vi "Online Spectrogram Monitoring (Sound Card).vi"() -> ()   [LabVIEW 2023]
doc: "This example shows how to configure a sound card device, continuously acquire sound data, and compute the real-time STFT spectrogram with the TFA Online STFT Spectrogram VI.\n\n<b>Instructions:</b>\n1) Run this VI.\n2) Speak or whistle into the microphone.\n3) Observe the <b>Spectrogram</b> to see the frequencies that this VI detects.\n4) Browse the Block Diagram of this example to learn how to configure the charts."
uses:
  <vilib>/sound2/lvsound2.llb/Sound Data Format.ctl
  <vilib>/Analysis/baseanly.llb/Mean (DBL).vi
  <vilib>/sound2/lvsound2.llb/Sound Input Read (DBL).vi
  <vilib>/addons/Time Frequency Analysis/Spectrogram.llb/TFA Online STFT Spectrogram (Real).vi
  <vilib>/addons/Time Frequency Analysis/_control.llb/TFA Configure Spectrogram Indicator (Predefined Color Table).vi
  <vilib>/addons/_Advanced Signal Processing/NI_AdvSigProcTFA.lvlib
  <vilib>/Analysis/NI_AALBase.lvlib
panel:
  out "aspt-left-top":bool
  in  "dB on?(F)":bool
  in  "Stop":bool
  out "Signal":dbl[](graph)
  out "Spectrogram":dbl[][](graph)
  # "Overview: Shows how to configure a sound card device, continuously acquire sound data, and compute the real-time STFT spectrogram with the TFA Online STFT Spectrogram VI.\nRequirements: LabVIEW Full Development System, Advanced Signal Processing Toolkit, microphone\nInstructions: \n1. Run this VI.\n2. Speak or whistle into the microphone.\n3. Observe the Spectrogram to see the frequencies that this VI detects.\n4. Browse the block diagram of this example to learn how to configure the charts.\n5. Click Stop to stop the VI."
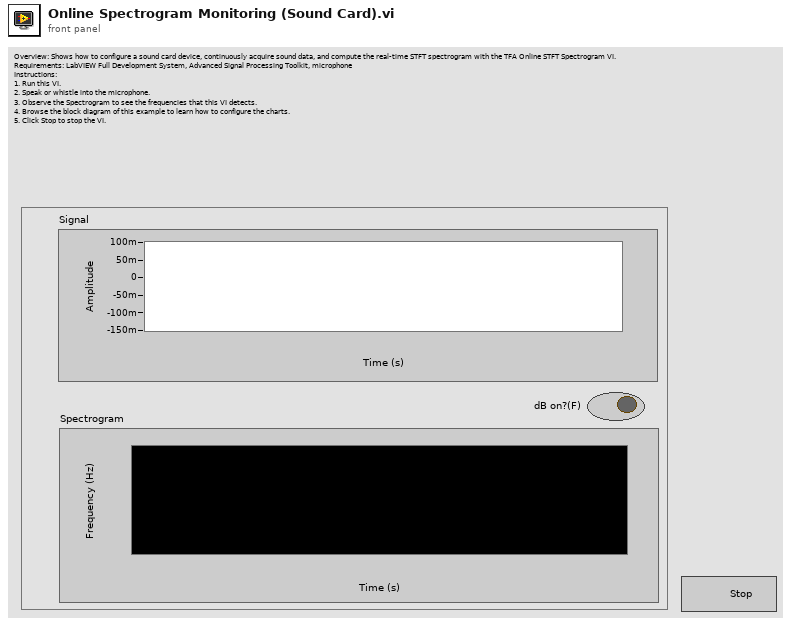
[diagram p1: front panel]
types:
  T1 = typedef "Sound Data Format.ctl" = cluster{"sample rate (S/s)":dbl, "number of channels":i32, "bits per sample":i32}
  T2 = typedef "Sound Input Task ID.ctl" = u32
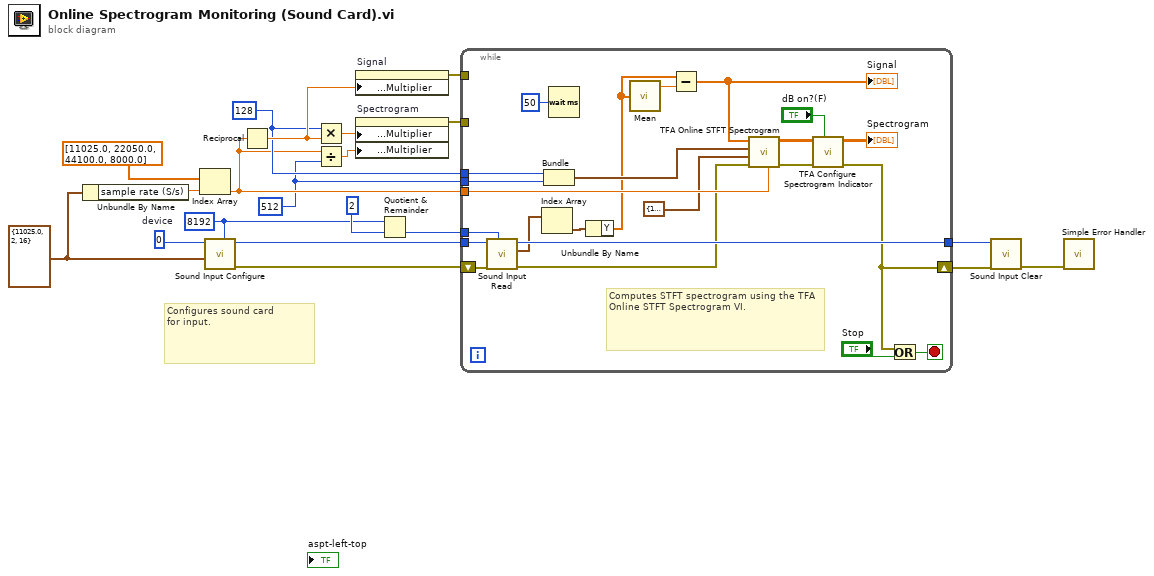
[diagram p0: block diagram]
diagram:
  w8 = T1 {"sample rate (S/s)"=11025.0, "number of channels"=2, "bits per sample"=16} ("sound format")
  w9 = 512 ("FFT block size")
  w12 = 128 ("Step size")
  w4 = 8192 ("Buffer Size")
  w20 = u32 0  # device
  # "Configures sound card\nfor input."
  n1 = Unbundle By Name(w8) -> ("sample rate (S/s)"=w17:dbl)
  n2 = Index Array(array=dbl[] [11025.0, 22050.0, 44100.0, 8000.0], index=w17) -> (element=w10:dbl)
  n3 = call <vilib>:"Sound Input Configure.vi"("number of samples/ch"=w4, "sound format"=w8, "device ID"=w20) -> ("error out"=w6:errorcluster, "task ID"=w7:T2)  [unwired: 7 in]
  n4 = Reciprocal(x=w10) -> (1/x=w16:dbl)
  n5 = Multiply(x=w12, y=w16) -> (x*y=w13:dbl)
  n6 = Divide(x=w10, y=w9) -> (x/y=w11:dbl)
  n7 = property on="Signal" class="WFChart (strict)"("X Scale.Offset and Multiplier:Multiplier"=w16) -> (error out=w14:errorcluster)  [unwired: 2 in, 1 out]
  n8 = property on="Spectrogram" class="IntChart (strict)"("X Scale.Offset and Multiplier:Multiplier"=w13, "Y Scale.Offset and Multiplier:Multiplier"=w11) -> (error out=w15:errorcluster)  [unwired: 2 in, 1 out]
  n9 = Quotient & Remainder(x=w4, y=2) -> (floor(x/y)=w3:i32)  [unwired: 1 out]
  n10 = while {
    shift-left: w6 -> [w39]
    shift-right: [w26] -> w1
    tunnel: [w43] -> w2
    tunnel: w7 -> [w40]
    tunnel: w10 -> [w38]
    tunnel: w15 -> [_]
    tunnel: w14 -> [_]
    tunnel: w12 -> [w34]
    tunnel: w9 -> [w33]
    tunnel: w3 -> [w21]
    stop <- w41 stop-if-true
    # "Computes STFT spectrogram using the TFA Online STFT Spectrogram VI."
    n11 = call-poly <vilib>:"Sound Input Read.vi"("number of samples/ch"=w21, "error in (no error)"=w39, "task ID"=w40) -> ("error out"=w27:errorcluster, "data"=w24:waveform(dbl)[], "task ID out"=w43:T2)  [unwired: 6 in]
    n12 = Index Array(array=w24) -> (element=w23:waveform(dbl))  [unwired: 1 in]
    n13 = Bundle("Step size"=w34, "FFT block size"=w33) -> (w37:cluster{"Step size":i32, "FFT block size":i32})  [unwired: 1 out]
    n14 = Wait (ms)(milliseconds to wait=u32 50) -> ()  [unwired: 1 out]
    n15 = Unbundle By Name(w23) -> ("Y"=w22:dbl[])
    n16 = call-poly <vilib>:"Mean.vi"("X"=w22) -> ("mean"=w36:dbl)  [unwired: 1 out]
    n17 = Subtract(x=w22, y=w36) -> (x-y=w35:dbl[])
    "Signal" <- w35
    n18 = call-poly <vilib>:"TFA Online STFT Spectrogram.vi"("sampling rate"=w38, "error in (no error)"=w27, "window info"=cluster{"type":i32, "length":i32} {"type"=1, "length"=512}, "time-frequency sampling info"=w37, "signal"=w35) -> ("error out"=w25:errorcluster, "spectrogram"=w32:dbl[][])  [unwired: 1 in, 4 out]
    n19 = call-poly <vilib>:"TFA Configure Spectrogram Indicator.vi"("dB on? (F)"="dB on?(F)", "error in (no error)"=w25, "spectrogram"=w32) -> ("error out"=w26:errorcluster, "TF spectrogram indicator"=→"Spectrogram":dbl[][])  [unwired: 4 in, 3 out]
    n20 = Or(x=w26, y="Stop") -> (x .or. y?=w41:bool)
  }
  n21 = call <vilib>:"Sound Input Clear.vi"("error in (no error)"=w1, "task ID"=w2) -> ("error out"=w19:errorcluster)  [unwired: 9 in]
  n22 = call <vilib>:"Simple Error Handler.vi"("error in (no error)"=w19) -> ()  [unwired: 4 in, 5 out]
